vi "Parse One String.vi"(10 "State String":string) -> (2 "Argument":string)   [LabVIEW 2013]
doc: "This sub-VI parses a single string argument from an input string of the format \"state:argument\"."
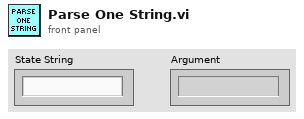
[diagram p1: front panel]
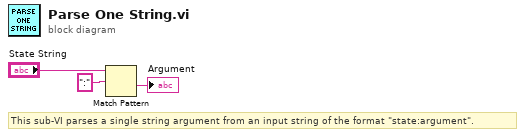
[diagram p0: block diagram]
diagram:
  # "This sub-VI parses a single string argument from an input string of the format \"state:argument\"."
  n1 = Match Pattern(string="State String", regular expression=":") -> (after substring=→"Argument":string)  [unwired: 1 in, 3 out]
